vi "UHR-Fleezers Control (host) - 12.6.vi"() -> ()   [LabVIEW 2012] (continued)
                          n988 = call <vilib>:"Beep.vi"() -> ()  [unwired: 3 in, 9 out]
                          n989 = local write "Waiting"(FALSE ("Waiting")) -> ()
                          n990 = Increment(x=w1498) -> (x+1=w1497:u8)
                          n991 = case shown="\"Yank\"" w1500 {
                            tunnel: w1497 -> [_ _ w1507]
                            frame "Image" {
                              n992 = property on="Confocal Image" class="Bool (strict)"("Val(Sgnl)"=TRUE ("Value (Signaling)")) -> ()  [unwired: 2 in, 2 out]
                            }
                            frame "Alarm", Default {
                            }
                            frame "Yank" {
                              n993 = flat-sequence {
                                tunnel: w1507 -> [w1510]
                                tunnel: [w1509] -> w1506
                                tunnel: ["N Array El"] -> w1505
                                tunnel: w1506 -> [w1524]
                                tunnel: w1505 -> [w1520]
                                frame #0 {
                                n994 = Multiply(x="Yank Delay (s)", y=1000.0) -> (x*y=w1513:dbl)
                                n995 = Quotient & Remainder(x=w1510, y="N Array El") -> (x-y*floor(x/y)=w1509:u8)  [unwired: 1 out]
                                n996 = Wait (ms)(milliseconds to wait=w1513) -> ()  [unwired: 1 out]
                                }
                                frame #1 {
                                n997 = Random Number (0-1)() -> (number: 0 to 1=w1521:dbl)
                                n998 = Multiply(x=w1520, y=w1521) -> (x*y=w1519:dbl)
                                n999 = Round Toward -Infinity(1:w1519) -> (0:w1518:dbl)
                                n1000 = Select(t=w1518, s="Random Choice", f=w1524) -> (s? t:f=w1522:dbl)
                                n1001 = Select(t="Yank to Trap Delta (MHz)", s="Yank to which?", f="Yank to SP") -> (s? t:f=w1515:dbl[])
                                n1002 = Index Array(array=w1515, index=w1522) -> (element=w1525:dbl)
                                n1003 = case shown="False" "Yank to which?" {
                                tunnel: w1525 -> [w1526 w1552]
                                frame False {
                                n1004 = flat-sequence {
                                tunnel: w1526 -> [w1527]
                                frame #0 {
                                n1005 = property on="Trap Pos FB SP" class="DigNum (strict)"("Val(Sgnl)"=w1527) -> ()  [unwired: 2 in, 2 out]
                                }
                                frame #1 {
                                n1006 = Wait (ms)(milliseconds to wait=u32 700) -> ()  [unwired: 1 out]
                                }
                                frame #2 {
                                n1007 = local read "Action (%)"() -> (w1532:dbl)
                                n1008 = Absolute Value(x=w1532) -> (abs(x)=w1531:dbl)
                                n1009 = Greater?(x=w1531, y=70.0) -> (0:w1529:bool)
                                n1010 = property on="Remove Action Offset" class="Bool (strict)"("Val(Sgnl)"=w1529) -> ()  [unwired: 2 in, 2 out]
                                }
                                frame #3 {
                                n1011 = for {
                                N: 4 -> [_]
                                n1012 = flat-sequence {
                                frame #0 {
                                n1013 = Wait (ms)(milliseconds to wait=u32 500) -> ()  [unwired: 1 out]
                                }
                                frame #1 {
                                n1014 = local read "Action (%)"() -> (w1538:dbl)
                                n1015 = Absolute Value(x=w1538) -> (abs(x)=w1537:dbl)
                                n1016 = Greater?(x=w1537, y=70.0) -> (0:w1535:bool)
                                n1017 = property on="Remove Action Offset" class="Bool (strict)"("Val(Sgnl)"=w1535) -> ()  [unwired: 2 in, 2 out]
                                }
                                }
                                }
                                }
                                frame #4 {
                                n1018 = local read "Shift confocal"() -> (w1542:bool)
                                n1019 = local read "Mean"() -> (w1545:dbl)
                                n1020 = Greater?(x=w1545, y=11.0) -> (0:w1541:bool)
                                n1021 = Not(x=w1541) -> (.not. x?=w1540:bool)
                                n1022 = And(x=w1540, y=w1542) -> (x .and. y?=w1539:bool)
                                n1023 = And(x=w1541, y=w1542) -> (x .and. y?=w1543:bool)
                                n1024 = case shown="True" w1543 {
                                frame False {
                                }
                                frame True {
                                n1025 = local read "Confocal X 2 (V)"() -> (w1548:dbl)
                                n1026 = local read "Confocal Y 2 (V)"() -> (w1549:dbl)
                                n1027 = property on="AO2" class="Slide (strict)"("Val(Sgnl)"=w1548) -> ()  [unwired: 2 in, 2 out]
                                n1028 = property on="AO1" class="Slide (strict)"("Val(Sgnl)"=w1549) -> ()  [unwired: 2 in, 2 out]
                                }
                                }
                                n1029 = case shown="True" w1539 {
                                frame False {
                                }
                                frame True {
                                n1030 = local read "Confocal X 1 (V)"() -> (w1546:dbl)
                                n1031 = local read "Confocal Y 1 (V)"() -> (w1547:dbl)
                                n1032 = property on="AO1" class="Slide (strict)"("Val(Sgnl)"=w1547) -> ()  [unwired: 2 in, 2 out]
                                n1033 = property on="AO2" class="Slide (strict)"("Val(Sgnl)"=w1546) -> ()  [unwired: 2 in, 2 out]
                                }
                                }
                                }
                                frame #5 {
                                n1034 = Wait (ms)(milliseconds to wait=u32 1500) -> ()  [unwired: 1 out]
                                }
                                frame #6 {
                                n1035 = property on="Rem fb disp offset" class="Bool (strict)"("Val(Sgnl)"=TRUE ("Value (Signaling)")) -> ()  [unwired: 2 in, 2 out]
                                }
                                }
                                }
                                frame True {
                                n1036 = flat-sequence {
                                tunnel: w1552 -> [w1553]
                                frame #0 {
                                n1037 = property on="Trap Delta (MHz)" class="DigNum (strict)"("Val(Sgnl)"=w1553) -> ()  [unwired: 2 in, 2 out]
                                }
                                frame #1 {
                                n1038 = Wait (ms)(milliseconds to wait=u32 500) -> ()  [unwired: 1 out]
                                }
                                frame #2 {
                                n1039 = local read "Shift confocal"() -> (w1557:bool)
                                n1040 = local read "Mean"() -> (w1555:dbl)
                                n1041 = Greater?(x=w1555, y=11.0) -> (0:w1558:bool)
                                n1042 = Not(x=w1558) -> (.not. x?=w1559:bool)
                                n1043 = And(x=w1559, y=w1557) -> (x .and. y?=w1561:bool)
                                n1044 = And(x=w1558, y=w1557) -> (x .and. y?=w1560:bool)
                                n1045 = case shown="True" w1560 {
                                frame False {
                                }
                                frame True {
                                n1046 = local read "Confocal Y 2 (V)"() -> (w1565:dbl)
                                n1047 = local read "Confocal X 2 (V)"() -> (w1564:dbl)
                                n1048 = property on="AO1" class="Slide (strict)"("Val(Sgnl)"=w1565) -> ()  [unwired: 2 in, 2 out]
                                n1049 = property on="AO2" class="Slide (strict)"("Val(Sgnl)"=w1564) -> ()  [unwired: 2 in, 2 out]
                                }
                                }
                                n1050 = case shown="True" w1561 {
                                frame False {
                                }
                                frame True {
                                n1051 = local read "Confocal X 1 (V)"() -> (w1562:dbl)
                                n1052 = local read "Confocal Y 1 (V)"() -> (w1563:dbl)
                                n1053 = property on="AO2" class="Slide (strict)"("Val(Sgnl)"=w1562) -> ()  [unwired: 2 in, 2 out]
                                n1054 = property on="AO1" class="Slide (strict)"("Val(Sgnl)"=w1563) -> ()  [unwired: 2 in, 2 out]
                                }
                                }
                                }
                                }
                                }
                                }
                                }
                              }
                            }
                          }
                          n1055 = local read "Time (s)"() -> (w1499:dbl)
                          "Fl. High" <- TRUE ("Yanking")
                        }
                        frame #1 {
                          n1056 = local read "Auto F Reset"() -> (w1566:bool)
                          n1057 = case shown="True" w1566 {
                            tunnel: w1571 -> [_ w1575]
                            tunnel: w1570 -> [_ w1574]
                            tunnel: w1569 -> [_ w1573]
                            tunnel: w1567 -> [_ w1572]
                            frame False {
                            }
                            frame True {
                              n1058 = node-c288() -> (w1577:T23)  [unwired: 4 out]
                              n1059 = timed-loop {
                                timing: w1577 -> [_]
                                timing-out: [_] -> w1576
                                tunnel: w1575 -> [w1595]
                                tunnel: w1574 -> [w1594]
                                tunnel: w1573 -> [w1593]
                                tunnel: w1572 -> [w1592]
                                stop <- w1578 stop-if-true
                                n1060 = node-c288() -> ()  [unwired: 2 out]
                                n1061 = local read "Fl. Delta Thresh. (kHz)"() -> (w1586:dbl)
                                n1062 = local read "Fl. Triggered..."() -> (w1591:bool)
                                n1063 = local read "Delta Fl. 1"() -> (w1582:dbl)
                                n1064 = local read "Delta Fl. 2"() -> (w1580:dbl)
                                n1065 = local read "Stop All"() -> (w1589:bool)
                                n1066 = local read "APD to Watch"() -> (w1581:bool)
                                n1067 = Select(t=w1582, s=w1581, f=w1580) -> (s? t:f=w1579:dbl)
                                n1068 = Not(x=w1591) -> (.not. x?=w1590:bool)
                                n1069 = Multiply(x=w1586, y=1000.0) -> (x*y=w1585:dbl)
                                n1070 = Negate(x=w1585) -> (-x=w1584:dbl)
                                n1071 = Less?(x=w1579, y=w1584) -> (x < y?=w1588:bool)
                                n1072 = Compound Arithmetic op=OR(w1588, w1589, w1590, "Reset Force") -> (w1578:bool)
                                n1073 = case shown="True" w1578 {
                                tunnel: w1595 -> [_ w1610]
                                tunnel: w1594 -> [_ w1609]
                                tunnel: w1593 -> [_ w1599]
                                tunnel: w1592 -> [_ w1601]
                                frame False {
                                }
                                frame True {
                                n1074 = local read "Time (s)"() -> (w1600:dbl)
                                n1075 = case shown="\"Yank\"" w1609 {
                                tunnel: w1610 -> [_ w1613]
                                tunnel: w1601 -> [_ w1611]
                                frame "Image", Default {
                                }
                                frame "Yank" {
                                n1076 = flat-sequence {
                                tunnel: [w1619] -> w1614
                                tunnel: w1613 -> [w1619]
                                tunnel: [w1615] -> w1612
                                tunnel: w1611 -> [w1615]
                                tunnel: w1614 -> [w1622]
                                tunnel: w1612 -> [w1620]
                                frame #0 {
                                n1077 = local read "Yank Delay (s)"() -> (w1618:dbl)
                                n1078 = Multiply(x=w1618, y=1000.0) -> (x*y=w1616:dbl)
                                n1079 = Wait (ms)(milliseconds to wait=w1616) -> ()  [unwired: 1 out]
                                }
                                frame #1 {
                                n1080 = local read "Yank to which?"() -> (w1621:bool)
                                n1081 = case shown="False" w1621 {
                                tunnel: w1622 -> [_ w1649]
                                tunnel: w1620 -> [w1623 _]
                                frame False {
                                n1082 = flat-sequence {
                                tunnel: w1623 -> [w1624]
                                frame #0 {
                                n1083 = property on="Trap Pos FB SP" class="DigNum (strict)"("Val(Sgnl)"=w1624) -> ()  [unwired: 2 in, 2 out]
                                }
                                frame #1 {
                                n1084 = Wait (ms)(milliseconds to wait=u32 700) -> ()  [unwired: 1 out]
                                }
                                frame #2 {
                                n1085 = local read "Action (%)"() -> (w1629:dbl)
                                n1086 = Absolute Value(x=w1629) -> (abs(x)=w1628:dbl)
                                n1087 = Greater?(x=w1628, y=70.0) -> (0:w1626:bool)
                                n1088 = property on="Remove Action Offset" class="Bool (strict)"("Val(Sgnl)"=w1626) -> ()  [unwired: 2 in, 2 out]
                                }
                                frame #3 {
                                n1089 = for {
                                N: 4 -> [_]
                                n1090 = flat-sequence {
                                frame #0 {
                                n1091 = Wait (ms)(milliseconds to wait=u32 500) -> ()  [unwired: 1 out]
                                }
                                frame #1 {
                                n1092 = local read "Action (%)"() -> (w1635:dbl)
                                n1093 = Absolute Value(x=w1635) -> (abs(x)=w1634:dbl)
                                n1094 = Greater?(x=w1634, y=70.0) -> (0:w1632:bool)
                                n1095 = property on="Remove Action Offset" class="Bool (strict)"("Val(Sgnl)"=w1632) -> ()  [unwired: 2 in, 2 out]
                                }
                                }
                                }
                                }
                                frame #4 {
                                n1096 = local read "Shift confocal"() -> (w1640:bool)
                                n1097 = local read "Mean"() -> (w1642:dbl)
                                n1098 = Greater?(x=w1642, y=11.0) -> (0:w1639:bool)
                                n1099 = Not(x=w1639) -> (.not. x?=w1638:bool)
                                n1100 = And(x=w1639, y=w1640) -> (x .and. y?=w1637:bool)
                                n1101 = And(x=w1638, y=w1640) -> (x .and. y?=w1636:bool)
                                n1102 = case shown="True" w1637 {
                                frame False {
                                }
                                frame True {
                                n1103 = local read "Confocal Y 2 (V)"() -> (w1646:dbl)
                                n1104 = local read "Confocal X 2 (V)"() -> (w1645:dbl)
                                n1105 = property on="AO2" class="Slide (strict)"("Val(Sgnl)"=w1645) -> ()  [unwired: 2 in, 2 out]
                                n1106 = property on="AO1" class="Slide (strict)"("Val(Sgnl)"=w1646) -> ()  [unwired: 2 in, 2 out]
                                }
                                }
                                n1107 = case shown="True" w1636 {
                                frame False {
                                }
                                frame True {
                                n1108 = local read "Confocal X 1 (V)"() -> (w1643:dbl)
                                n1109 = local read "Confocal Y 1 (V)"() -> (w1644:dbl)
                                n1110 = property on="AO1" class="Slide (strict)"("Val(Sgnl)"=w1644) -> ()  [unwired: 2 in, 2 out]
                                n1111 = property on="AO2" class="Slide (strict)"("Val(Sgnl)"=w1643) -> ()  [unwired: 2 in, 2 out]
                                }
                                }
                                }
                                frame #5 {
                                n1112 = Wait (ms)(milliseconds to wait=u32 1500) -> ()  [unwired: 1 out]
                                }
                                frame #6 {
                                n1113 = property on="Rem fb disp offset" class="Bool (strict)"("Val(Sgnl)"=TRUE ("Value (Signaling)")) -> ()  [unwired: 2 in, 2 out]
                                }
                                }
                                }
                                frame True {
                                n1114 = flat-sequence {
                                tunnel: w1649 -> [w1650]
                                frame #0 {
                                n1115 = property on="Trap Delta (MHz)" class="DigNum (strict)"("Val(Sgnl)"=w1650) -> ()  [unwired: 2 in, 2 out]
                                }
                                frame #1 {
                                n1116 = Wait (ms)(milliseconds to wait=u32 500) -> ()  [unwired: 1 out]
                                }
                                frame #2 {
                                n1117 = local read "Shift confocal"() -> (w1656:bool)
                                n1118 = local read "Mean"() -> (w1658:dbl)
                                n1119 = Greater?(x=w1658, y=11.0) -> (0:w1655:bool)
                                n1120 = Not(x=w1655) -> (.not. x?=w1654:bool)
                                n1121 = And(x=w1655, y=w1656) -> (x .and. y?=w1653:bool)
                                n1122 = And(x=w1654, y=w1656) -> (x .and. y?=w1652:bool)
                                n1123 = case shown="True" w1653 {
                                frame False {
                                }
                                frame True {
                                n1124 = local read "Confocal Y 2 (V)"() -> (w1662:dbl)
                                n1125 = local read "Confocal X 2 (V)"() -> (w1661:dbl)
                                n1126 = property on="AO2" class="Slide (strict)"("Val(Sgnl)"=w1661) -> ()  [unwired: 2 in, 2 out]
                                n1127 = property on="AO1" class="Slide (strict)"("Val(Sgnl)"=w1662) -> ()  [unwired: 2 in, 2 out]
                                }
                                }
                                n1128 = case shown="True" w1652 {
                                frame False {
                                }
                                frame True {
                                n1129 = local read "Confocal Y 1 (V)"() -> (w1660:dbl)
                                n1130 = local read "Confocal X 1 (V)"() -> (w1659:dbl)
                                n1131 = property on="AO2" class="Slide (strict)"("Val(Sgnl)"=w1659) -> ()  [unwired: 2 in, 2 out]
                                n1132 = property on="AO1" class="Slide (strict)"("Val(Sgnl)"=w1660) -> ()  [unwired: 2 in, 2 out]
                                }
                                }
                                }
                                }
                                }
                                }
                                }
                                }
                                }
                                }
                                n1133 = local read "Messages"() -> (w1608:string)
                                n1134 = Subtract(x=w1600, y=w1599) -> (x-y=w1606:dbl)
                                "Duration (s)" <- w1606
                                n1135 = Number To Decimal String(number=w1606, width (-)=i16 0) -> (decimal integer string=w1604:string)
                                n1136 = Concatenate Strings(w1604, " s fluorescence event." ("string")) -> (w1602:string)
                                n1137 = call "Update messages.vi"("Message to add"=w1602, "Old message string"=w1608) -> ("New message string"=w1607:string)
                                n1138 = local write "Reset Force"(FALSE ("Reset Force")) -> ()
                                n1139 = local write "Waiting"(TRUE ("Waiting")) -> ()
                                n1140 = local write "Messages"(w1607) -> ()
                                n1141 = local write "Fl. High"(FALSE ("Fl. High")) -> ()
                                n1142 = call <vilib>:"Beep.vi"() -> ()  [unwired: 3 in, 9 out]
                                }
                                }
                                n1143 = node-c288() -> ()  [unwired: 2 out]
                              }
                              n1144 = node-c288(w1576) -> ()  [unwired: 1 out]
                            }
                          }
                        }
                      }
                      n1145 = local read "Trap Delta (MHz)"() -> (w1491:dbl)
                      n1146 = local read "Trap Pos FB SP"() -> (w1486:fxp<+/-,16,1>)
                    }
                  }
                }
                frame #1 {
                  n1147 = local read "Stop All"() -> (w1672:bool)
                  n1148 = local read "Fl. Triggered..."() -> (w1670:bool)
                  n1149 = Not(x=w1670) -> (.not. x?=w1671:bool)
                  n1150 = Or(x=w1671, y=w1672) -> (x .or. y?=w1669:bool)
                }
              }
              n1151 = case shown="True" w1263 {
                frame False {
                }
                frame True {
                  n1152 = local read "Confocal Y 1 (V)"() -> (w1273:dbl)
                  n1153 = local read "Confocal X 1 (V)"() -> (w1272:dbl)
                  n1154 = property on="AO2" class="Slide (strict)"("Val(Sgnl)"=w1272) -> ()  [unwired: 2 in, 2 out]
                  n1155 = property on="AO1" class="Slide (strict)"("Val(Sgnl)"=w1273) -> ()  [unwired: 2 in, 2 out]
                }
              }
              n1156 = case shown="True" w1263 {
                frame False {
                }
                frame True {
                  w1271 = FALSE ("Fl. High")
                  n1157 = local write "Waiting"(w1271) -> ()
                  n1158 = local write "Fl. High"(w1271) -> ()
                }
              }
              n1159 = node-c288() -> ()  [unwired: 2 out]
            }
            n1160 = node-c288(w1261) -> ()  [unwired: 1 out]
          }
        }
      }
      event "Stop All": Value Change {
        n1161 = event-data() -> ()  [unwired: 7 out]
        n1162 = local read "Stop All"() -> (w1677:bool)
      }
    }
    n1163 = node-c288() -> ()  [unwired: 2 out]
  }
  n1164 = timed-loop "Basic control parameters (all FPGA settings, other basic controls)" {
    tunnel: w16 -> [w1686]
    shift-right: [w1685] -> _
    shift-left: errorcluster {"status"=FALSE, "code"=0, "source"=""} ("error out") -> [w1684]
    tunnel: [w1683] -> _
    timing: w126 -> [_]
    timing-out: [_] -> w125
    tunnel: w99 -> [w1682]
    tunnel: w71 -> [w1681]
    tunnel: w70 -> [w1680]
    tunnel: w69 -> [w1679]
    tunnel: w68 -> [w1678]
    stop <- w1683 stop-if-true
    n1165 = node-c288() -> ()  [unwired: 2 out]
    n1166 = event shown="[4] \"Phase adj. (AI1)\", \"+ phase (AI1)\", \"- phase (AI1)\": Value Change" {
      selector: _ -> [_ _ _ _ _ _ _ _ _ _ _ _ _ _ _ _ _ _ _ _ _ _ _ _ _ _ _ _ _ _ _ _ _ _ _ _ _ _ _ _ _ _ _ _ _ _ _ _ _ _ _ _ _ _ _ _ _ _ _ _ _ _ _ _ _ _ _ _ _ _ _ _ _ _]
      dyn-events: _ -> [_ _ _ _ _ _ _ _ _ _ _ _ _ _ _ _ _ _ _ _ _ _ _ _ _ _ _ _ _ _ _ _ _ _ _ _ _ _ _ _ _ _ _ _ _ _ _ _ _ _ _ _ _ _ _ _ _ _ _ _ _ _ _ _ _ _ _ _ _ _ _ _ _ _]
      timeout: _ -> [_ _ _ _ _ _ _ _ _ _ _ _ _ _ _ _ _ _ _ _ _ _ _ _ _ _ _ _ _ _ _ _ _ _ _ _ _ _ _ _ _ _ _ _ _ _ _ _ _ _ _ _ _ _ _ _ _ _ _ _ _ _ _ _ _ _ _ _ _ _ _ _ _ _]
      tunnel: w1686 -> [w1727 _ _ _ w1765 _ w1787 _ _ _ _ w1853 _ _ w1896 w1902 w1909 w1914 w1987 _ w2003 w2028 w2049 w2070 w2090 w2119 w2145 w2148 w2152 w2247 w2252 w2290 _ w2325 w2329 w2340 w2344 w2348 _ w2356 _ _ _ _ _ _ _ _ _ _ _ _ _ _ _ _ _ w2734 _ w2751 _ w2758 w2776 _ w2783 w2791 w2806 w2822 w2828 _ w2837 _ w2856 _]
      tunnel: [w1726 _ _ _ w1755 _ w1786 _ _ w1818 _ w1832 _ _ w1895 w1898 w1908 w1911 w1981 _ w2002 w2027 w2047 w2068 w2088 w2113 w2143 _ w2150 w2245 w2250 w2288 _ w2323 w2327 w2331 w2342 w2346 _ w2354 _ _ _ _ _ _ _ _ _ _ _ _ _ _ _ _ _ w2732 _ _ _ _ w2773 _ _ _ _ _ _ _ _ _ _ _] -> w1685
      tunnel: w1684 -> [w1725 _ _ _ w1764 _ w1785 _ _ w1818 _ w1852 _ _ w1894 w1897 w1907 w1910 w1986 _ w2001 w2026 w2048 w2069 w2089 w2118 w2144 w2147 w2151 w2246 w2251 w2289 _ w2324 w2328 w2339 w2343 w2347 _ w2355 _ _ _ _ _ _ _ _ _ _ _ _ _ _ _ _ _ w2733 _ w2750 _ w2757 w2775 _ w2782 w2790 w2805 w2821 w2827 _ w2836 _ w2855 _]
      tunnel: [_ _ _ _ _ _ _ _ _ w1817 _ _ _ _ _ _ _ _ _ _ _ _ _ _ _ _ _ _ _ _ _ _ _ _ _ _ _ _ _ _ _ _ _ _ _ _ _ _ _ _ _ _ _ _ _ _ _ _ _ _ _ _ _ _ _ _ _ _ _ _ _ _ _ _] -> w1683
      tunnel: [_ _ _ _ _ _ _ "Round T1 X" _ _ _ _ _ _ _ _ _ _ _ _ _ _ _ _ _ _ _ _ _ _ _ _ _ _ _ _ _ _ _ _ _ _ _ _ _ _ _ _ _ _ _ _ _ _ _ _ _ _ _ _ _ _ _ _ _ _ _ _ _ _ _ _ _ _] -> _
      tunnel: [_ _ _ "Adjust Scale\nto Mean" _ _ _ _ _ _ _ _ _ _ _ _ _ _ _ _ _ _ _ _ _ _ _ _ "Test ttrig" _ _ _ _ _ _ _ _ _ _ _ _ _ _ _ _ _ _ "Flush Sample" "Flush Pump 3" "Flush Pump 1" "Clear Volume" _ _ _ _ _ _ _ _ _ _ _ _ _ _ _ _ _ _ _ _ _ _ _] -> _
      tunnel: [_ _ _ _ _ _ _ _ "Round T2 X" _ "Delayed Interlace Start" _ _ _ _ _ _ _ _ _ _ _ _ _ _ _ _ _ _ _ _ _ _ _ _ _ _ _ _ _ _ _ _ _ _ _ _ _ _ _ _ _ _ _ _ _ _ _ _ _ _ _ _ _ _ _ _ _ _ _ _ _ _ _] -> _
      tunnel: w1682 -> [_ _ _ _ _ _ _ _ _ _ _ _ _ _ _ _ _ _ _ _ _ _ _ _ _ _ _ _ _ _ _ _ _ _ _ _ _ _ _ _ _ _ _ w2513 w2520 w2527 w2532 w2541 _ _ w2647 _ _ _ _ _ _ _ _ _ _ _ _ _ _ _ _ _ _ _ _ _ _ _]
      tunnel: w1681 -> [_ _ _ _ _ _ _ _ _ _ _ _ _ _ _ _ _ _ _ _ _ _ _ _ _ _ _ _ _ _ _ _ _ _ _ _ _ _ _ _ _ w2430 _ _ _ _ _ _ w2585 _ _ w2653 _ w2662 _ w2676 _ _ _ _ _ _ _ _ _ _ _ _ _ _ _ _ _ _]
      tunnel: w1680 -> [_ _ _ _ _ _ _ _ _ _ _ _ _ _ _ _ _ _ _ _ _ _ _ _ _ _ _ _ _ _ _ _ _ _ _ _ _ _ _ _ _ _ _ _ _ _ _ _ _ _ _ _ _ _ _ _ _ _ _ _ _ _ _ _ _ _ _ _ _ _ _ _ _ _]
      tunnel: w1679 -> [_ _ _ _ _ _ _ _ _ _ _ _ _ _ _ _ _ _ _ _ _ _ _ _ _ _ _ _ _ _ _ _ _ _ _ _ _ _ _ _ w2367 _ _ _ _ _ _ _ _ w2615 _ _ w2658 _ w2669 _ w2701 _ _ _ _ _ _ _ _ _ _ _ _ _ _ _ _ _]
      tunnel: w1678 -> [_ _ _ _ _ _ _ _ _ _ _ _ _ _ _ _ _ _ _ _ _ _ _ _ _ _ _ _ _ _ _ _ _ _ _ _ _ _ _ _ _ _ _ _ _ _ _ _ _ _ _ _ _ _ _ _ _ _ _ _ _ _ _ _ _ _ _ _ _ _ _ _ _ _]
      event "AI Count (ticks)", "Sets to FIFO (Traps)", "Save ave N", "FPGA Ave.", "# Samples/channel", "N sets to save": Value Change {
        # "So that if 'Save ave N' is updated, the AOD scanning code updates too."
        n1167 = event-data() -> ()  [unwired: 6 out]
        n1168 = local read "AI Count (ticks)"() -> (w1709:u16)
        n1169 = Unbundle By Name("Sets to FIFO (Traps)") -> ("Set 1"=w1692:bool, "Set 2"=w1691:bool, "Set 3"=w1690:bool)
        n1170 = Boolean To (0,1)(Boolean="Sets to FIFO (Traps)") -> (0, 1=w1717:cluster{"Set 1":i16, "Set 2":i16, "Set 3":i16})
        n1171 = xnode "Read/Write Control"("FPGA VI Reference In"=w1727, "error in"=w1725, "ai count"=w1709, "Set 1"=w1692, "Set 2"=w1691, "Set 3"=w1690, "N of AI1 Int Acq Sets"="N Acq Sets (Traps + Fl.)") -> ("error out"=w1726:errorcluster)  [unwired: 1 out]
        n1172 = Cluster To Array(cluster=w1717) -> (array=w1716:i16[])
        n1173 = To Unsigned Long Integer(number=w1716) -> (unsigned 32bit integer=w1698:u32[])
        n1174 = local read "Scan steps (AOD)"() -> (w1718:u64)
        n1175 = Multiply(x=w1709, y="N Acq Sets (Traps + Fl.)") -> (x*y=w1707:u16)
        n1176 = Divide(x=40000000.0, y=w1709) -> (x/y=w1701:dbl)
        "AI rate (Hz)" <- w1701
        "Ave. Rate (Hz)" <- w1701
        n1177 = Add Array Elements(numeric array=w1698) -> (sum=w1710:u32)
        "Trap Sets" <- w1710
        n1178 = Reciprocal(x=w1701) -> (1/x=→"Ave. Period (s)":dbl)
        n1179 = property on="Scan steps (AOD)" class="DigNum (strict)"("Val(Sgnl)"=w1718) -> ()  [unwired: 2 in, 2 out]
        n1180 = Divide(x=w1701, y="N Acq Sets (Traps + Fl.)") -> (x/y=w1722:dbl)
        "Data Rate (Hz)" <- w1722
        n1181 = Reciprocal(x=w1722) -> (1/x=→"Data Period (s)":dbl)
        n1182 = local read "Save ave N"() -> (w1721:dbl)
        n1183 = Divide(x=w1722, y=w1721) -> (x/y=w1720:dbl)
        "Save Data Rate (Hz)" <- w1720
        n1184 = Reciprocal(x=w1720) -> (1/x=→"Save Data Period (s)":dbl)
        n1185 = Multiply(x=w1707, y="# Samples/trap") -> (x*y=w1705:u32)
        "Counts/DMA" <- w1705
        n1186 = property on="Trap Disp. Downsample" class="DigNum (strict)"("Maximum"="# Samples/trap") -> ()  [unwired: 2 in, 2 out]
        n1187 = Multiply(x=w1710, y="# Samples/trap") -> (x*y=w1699:u32)
        "# Samples/channel" <- w1699
        n1188 = Multiply(x=w1699, y=u32 8) -> (x*y=→"Trap AI Elements/DMA read":u32)
        n1189 = local read "APD Int. Count"() -> (w1706:u32)
        n1190 = Multiply(x=w1699, y=u32 3) -> (x*y=→"Trap Pos Elements/DMA read":u32)
        n1191 = Divide(x=w1705, y=w1706) -> (x/y=w1696:dbl)
        "APD Samples/FIFO Acq." <- w1696
        n1192 = Divide(x=w1705, y=40000000.0) -> (x/y=w1703:dbl)
        "DMA Update Period (s)" <- w1703
        n1193 = local read "Number of APDs"() -> (w1689:u8)
        n1194 = Multiply(x=w1689, y=w1696) -> (x*y=→"APD Elements/DMA read":dbl)
        n1195 = property on="APD Disp. Downsample" class="DigNum (strict)"("Maximum"=w1696) -> ()  [unwired: 2 in, 2 out]
        n1196 = local read "N sets to save"() -> (w1715:u32)
        n1197 = Multiply(x=w1703, y=w1715) -> (x*y=→"Total Time (s)":dbl)
        "FPGA Averaging" <- FALSE ("FPGA Averaging")
      }
      event "Remove Offset": Value Change {
        n1198 = event-data() -> ()  [unwired: 7 out]
        n1199 = local write "Remove Offset"(FALSE ("Remove Offset")) -> ()
        n1200 = local read "Bead Mean (nm)"() -> (w1729:dbl)
        n1201 = local read "Offset (nm)"() -> (w1730:dbl)
        n1202 = Add(x=w1729, y=w1730) -> (x+y=w1728:dbl)
        n1203 = local write "Offset (nm)"(w1728) -> ()
        n1204 = disable-structure shown="Disabled" {
          frame Disabled {
            n1205 = local read "Bead Mean (nm)"() -> (w1735:dbl)
            n1206 = Add(y=w1735) -> (x=w1734:dbl, x+y=w1733:dbl)
            n1207 = Subtract(x=w1735, y=w1734) -> (x-y=w1732:dbl)
            n1208 = property on="Bead Separation" class="WFChart (strict)"("YScale.Minimum"=w1732) -> ()  [unwired: 2 in, 2 out]
            n1209 = property on="Bead Separation" class="WFChart (strict)"("YScale.Maximum"=w1733) -> ()  [unwired: 2 in, 2 out]
          }
          frame Enabled {
          }
        }
      }
      event "Detector Type": Value Change {
        n1210 = event-data() -> ()  [unwired: 7 out]
        n1211 = local read "AI labels"() -> (w1736:string[])
        n1212 = property on="High Res. Display" class="Ring (strict)"("Strings []"=w1736) -> ()  [unwired: 2 in, 2 out]
        n1213 = Build Array (concatenate)(w1736, "none") -> (w1737:string[])
        n1214 = property on="FFT 1 Choice 1" class="Ring (strict)"("Strings []"=w1737) -> ()  [unwired: 2 in, 2 out]
        n1215 = property on="FFT 1 Choice 2" class="Ring (strict)"("Strings []"=w1737) -> ()  [unwired: 2 in, 2 out]
        n1216 = property on="FFT 2 Choice 1" class="Ring (strict)"("Strings []"=w1737) -> ()  [unwired: 2 in, 2 out]
        n1217 = property on="FFT 2 Choice 2" class="Ring (strict)"("Strings []"=w1737) -> ()  [unwired: 2 in, 2 out]
        n1218 = Bundle("APD 1", "APD 2") -> (w1740:cluster{string, string})  [unwired: 1 out]
        n1219 = Cluster To Array(cluster=w1740) -> (array=w1738:string[])
        n1220 = Build Array (concatenate)(w1738, w1737) -> (w1742:string[])
        n1221 = Array Size(array=w1742) -> (size(s)=w1743:i32)
        n1222 = property on="Signals to Plot" class="LstBox (strict)"("Item Names"=w1742) -> ()  [unwired: 2 in, 2 out]
        n1223 = property on="Signals to Plot" class="LstBox (strict)"("Number of Rows"=w1743) -> ()  [unwired: 2 in, 2 out]
        n1224 = property on="All Signals" class="WFChart (strict)"("LegNumRows"=w1743) -> ()  [unwired: 2 in, 2 out]
      }
      event "Adjust Scale\nto Mean": Value Change {
        n1225 = event-data() -> ()  [unwired: 7 out]
        n1226 = local read "APD 1 Rate (Hz)"() -> (w1752:dbl)
        n1227 = Multiply(x=1000.0, y="Above (kHz)") -> (x*y=w1750:dbl)
        n1228 = Multiply(x=1000.0, y="Below (kHz)") -> (x*y=w1748:dbl)
        n1229 = Add(x=w1750, y=w1752) -> (x+y=w1745:dbl)
        n1230 = Subtract(x=w1752, y=w1748) -> (x-y=w1746:dbl)
        n1231 = property on="APD Chart" class="WFChart (strict)"("YScale.Minimum"=w1746) -> ()  [unwired: 2 in, 2 out]
        n1232 = property on="APD Chart" class="WFChart (strict)"("YScale.Maximum"=w1745) -> ()  [unwired: 2 in, 2 out]
      }
      event "Phase adj. (AI1)", "+ phase (AI1)", "- phase (AI1)": Value Change {
        n1233 = event-data() -> ()  [unwired: 7 out]
        n1234 = Negate(x="Phase adj. (AI1)") -> (-x=w1762:i16)
        n1235 = Select(t=w1762, s="- phase (AI1)", f="Phase adj. (AI1)") -> (s? t:f=w1761:i16)
        n1236 = xnode "Read/Write Control"("FPGA VI Reference In"=w1765, "error in"=w1764, "Phase count adjustment"=w1761) -> ("FPGA VI Reference Out"=w1760:T20, "error out"=w1759:errorcluster)  [unwired: 1 in]
        n1237 = Or(x="- phase (AI1)", y="+ phase (AI1)") -> (x .or. y?=w1756:bool)
        n1238 = xnode "Read/Write Control"("FPGA VI Reference In"=w1760, "error in"=w1759, "+ phase"=w1756) -> ("error out"=w1755:errorcluster)  [unwired: 1 in, 1 out]
      }
      event "Signals to Plot": Double Click {
        w1768 = u32 9868950 ("Color Box")
        n1239 = event-data() -> ("Row"=w1770:i32)  [unwired: 9 out]
        n1240 = property on="All Signals" class="WFChart (strict)"("Active Plot"=w1770) -> (error out=w1781:errorcluster)  [unwired: 2 in, 1 out]
        n1241 = property on="All Signals" class="WFChart (strict)" props=["Plot", "Visible?", "Plot", "Plot Color"](error in=w1781) -> (error out=w1780:errorcluster, "Plot.Visible?"=w1779:bool)  [unwired: 1 in, 2 out]
        n1242 = Select(t=FALSE ("Plot.Visible"), s=w1779, f=TRUE ("Plot.Visible")) -> (s? t:f=w1774:bool)
        n1243 = property on="All Signals" class="WFChart (strict)"(error in=w1780, "Plot.Visible?"=w1774) -> (error out=w1776:errorcluster)  [unwired: 1 in, 1 out]
        n1244 = property on="All Signals" class="WFChart (strict)"(error in=w1776) -> (error out=w1771:errorcluster, "Plot.Plot Color"=w1775:u32)  [unwired: 1 in, 1 out]
        n1245 = property on="Signals to Plot" class="LstBox (strict)"(error in=w1771, "Active Row"=w1770) -> (error out=w1769:errorcluster)  [unwired: 1 in, 1 out]
        n1246 = Select(t=w1775, s=w1774, f=u32 0) -> (s? t:f=w1772:u32)
        n1247 = property on="Signals to Plot" class="LstBox (strict)"(error in=w1769, "CellFontColor"=w1772, "SelColor"=w1768, "CellBG"=w1768, "CellFontSize"=u32 20 ("Active Row:Cell Font:Size"), "CellFontBold"=TRUE ("Active Row:Cell Font:Bold")) -> ()  [unwired: 1 in, 2 out]
      }
      event "BD 1 Frequency 1 (MHz)", "BD 1 Frequency 2 (MHz)", "BD 1 Frequency 3 (MHz)", "BD 2 Frequency 1 (MHz)", "BD 2 Frequency 2 (MHz)", "BD 2 Frequency 3 (MHz)", "Trap Delta (MHz)": Value Change {
        n1248 = event-data() -> ("CtlRef"=w1784:refnum<vi>)  [unwired: 6 out]
        n1249 = control-ref of="Trap Delta (MHz)"() -> (w1783:refnum<vi>)
        n1250 = Equal?(x=w1783, y=w1784) -> (x = y?=w1782:bool)
        n1251 = case shown="False" "Oscillate Set 1" {
          tunnel: w1787 -> [w1807 _]
          tunnel: [w1806 w1810] -> w1786
          tunnel: w1785 -> [w1805 w1810]
          tunnel: w1782 -> [w1790 _]
          frame False {
            n1252 = local read "BD 1 Frequency 2 (MHz)"() -> (w1794:dbl)
            n1253 = local read "BD 1 Frequency 1 (MHz)"() -> (w1792:dbl)
            n1254 = Subtract(x=w1794, y="Trap Delta (MHz)") -> (x-y=w1791:dbl)
            n1255 = Select(t=w1791, s=w1790, f=w1792) -> (s? t:f=w1789:dbl)
            n1256 = local read "Y RF Frequency Limits (MHz)"() -> (w1795:T16)
            n1257 = local read "X RF Frequency Limits (MHz)"() -> (w1796:T16)
            n1258 = local read "BD 1 Frequency 3 (MHz)"() -> (w1808:dbl)
            n1259 = local write "BD 1 Frequency 1 (MHz)"(w1789) -> ()
            n1260 = local read "BD 2 Frequency 1 (MHz)"() -> (w1799:dbl)
            n1261 = local read "BD 2 Frequency 2 (MHz)"() -> (w1798:dbl)
            n1262 = local read "BD 2 Frequency 3 (MHz)"() -> (w1809:dbl)
            n1263 = call "set RF board frequency - interlace.vi"("Board 2 Frequency Limits"=w1795, "Board 1 Frequency Limits"=w1796, "error in"=w1805, "FPGA VI Reference In"=w1807, "Board 2 Frequency 3 (MHz)"=w1809, "Board 1 Frequency 3 (MHz)"=w1808, "Board 2 Frequency 2 (MHz)"=w1798, "Board 2 Frequency 1 (MHz)"=w1799, "Board 1 Frequency 2 (MHz)"=w1794, "Board 1 Frequency 1  (MHz)"=w1789) -> ("error out"=w1806:errorcluster)  [unwired: 1 out]
            n1264 = Subtract(x=w1799, y=w1798) -> (x-y=w1803:dbl)
            n1265 = Subtract(x=w1789, y=w1794) -> (x-y=w1804:dbl)
            n1266 = Square(x=w1803) -> (x^2=w1801:dbl)
            n1267 = Square(x=w1804) -> (x^2=w1802:dbl)
            n1268 = Add(x=w1802, y=w1801) -> (x+y=w1800:dbl)
            n1269 = Square Root(x=w1800) -> (sqrt(x)=w1797:dbl)
            n1270 = local write "Trap Delta (MHz)"(w1797) -> ()
            n1271 = property on="Initial delta (MHz)" class="DigNum (strict)"("Val(Sgnl)"=w1797) -> ()  [unwired: 2 in, 2 out]
          }
          frame True {
          }
        }
      }
      event "Round T1 X": Value Change {
        n1272 = event-data() -> ()  [unwired: 7 out]
        n1273 = local read "BD 1 Frequency 1 (MHz)"() -> (w1813:dbl)
        n1274 = Round To Nearest(number=w1813) -> (nearest integer value=w1812:dbl)
        n1275 = property on="BD 1 Frequency 1 (MHz)" class="DigNum (strict)"("Val(Sgnl)"=w1812) -> ()  [unwired: 2 in, 2 out]
      }
      event "Round T2 X": Value Change {
        n1276 = event-data() -> ()  [unwired: 7 out]
        n1277 = local read "BD 1 Frequency 2 (MHz)"() -> (w1815:dbl)
        n1278 = Round To Nearest(number=w1815) -> (nearest integer value=w1814:dbl)
        n1279 = property on="BD 1 Frequency 2 (MHz)" class="DigNum (strict)"("Val(Sgnl)"=w1814) -> ()  [unwired: 2 in, 2 out]
      }
      event "Stop All": Value Change {
        n1280 = event-data() -> ()  [unwired: 7 out]
        n1281 = local read "Stop All"() -> (w1817:bool)
      }
      event "Delayed Interlace Start": Value Change {
        n1282 = event-data() -> ()  [unwired: 7 out]
        n1283 = flat-sequence {
          frame #0 {
            n1284 = Multiply(x="Delay to Interlace (s)", y=1000.0) -> (x*y=w1820:dbl)
            n1285 = Wait (ms)(milliseconds to wait=w1820) -> ()  [unwired: 1 out]
          }
          frame #1 {
            n1286 = property on="Laser interlacing mode" class="RadioBtnsControl (strict)"("Val(Sgnl)"=enum32{"Laser ON", "Laser OFF", "Interlace"}."Interlace" ("Value (Signaling)")) -> ()  [unwired: 2 in, 2 out]
          }
        }
      }
      event "BD 1 Amplitude 1 (%)", "BD 1 Amplitude 2 (%)", "BD 1 Amplitude 3 (%)", "BD 2 Amplitude 1 (%)", "BD 2 Amplitude 2 (%)", "BD 2 Amplitude 3 (%)", "Trap 1 ON", "Trap 2 ON", "Trap 3 ON", "Feedback On/Off", "All FB On/Off": Value Change {
        w1844 = i16 1 ("f")
        n1287 = event-data() -> ()  [unwired: 7 out]
        n1288 = local write "Trap 1 (ON/OFF)"("Trap 1 ON") -> ()
        n1289 = local write "Trap 2 (ON/OFF)"("Trap 2 ON") -> ()
        n1290 = Boolean To (0,1)(Boolean="Trap 3 ON") -> (0, 1=w1845:i16)
        n1291 = Boolean To (0,1)(Boolean="Trap 1 ON") -> (0, 1=w1846:i16)
        n1292 = Boolean To (0,1)(Boolean="Trap 2 ON") -> (0, 1=w1847:i16)
        n1293 = Select(t=w1847, s="Trap ON/OFF X or Y Amp?", f=w1844) -> (s? t:f=w1842:i16)
        n1294 = Select(t=w1846, s="Trap ON/OFF X or Y Amp?", f=w1844) -> (s? t:f=w1843:i16)
        n1295 = Select(t=w1845, s="Trap ON/OFF X or Y Amp?", f=w1844) -> (s? t:f=w1841:i16)
        n1296 = Select(t=w1844, s="Trap ON/OFF X or Y Amp?", f=w1847) -> (s? t:f=w1839:i16)
        n1297 = Select(t=w1844, s="Trap ON/OFF X or Y Amp?", f=w1846) -> (s? t:f=w1840:i16)
        n1298 = Select(t=w1844, s="Trap ON/OFF X or Y Amp?", f=w1845) -> (s? t:f=w1838:i16)
        n1299 = And(x="All FB On/Off", y="Feedback On/Off") -> (x .and. y?=w1836:cluster{"Set 1":bool, "Set 2":bool})
        n1300 = local read "BD 1 Amplitude 1 (%)"() -> (w1856:dbl)
        n1301 = local read "BD 1 Amplitude 2 (%)"() -> (w1855:dbl)
        n1302 = local read "BD 1 Amplitude 3 (%)"() -> (w1854:dbl)
        n1303 = Unbundle By Name(w1836) -> ("Set 1"=w1831:bool, "Set 2"=w1828:bool)
        n1304 = local read "Y RF Amplitude Limits (%)"() -> (w1824:T16)
        n1305 = local read "X RF Amplitude Limits (%)"() -> (w1825:T16)
        n1306 = local read "BD 2 Amplitude 1 (%)"() -> (w1857:dbl)
        n1307 = local read "BD 2 Amplitude 2 (%)"() -> (w1858:dbl)
        n1308 = local read "BD 2 Amplitude 3 (%)"() -> (w1859:dbl)
        n1309 = And(x="Trap 2 ON", y=w1828) -> (x .and. y?=w1826:bool)
        n1310 = And(x="Trap 1 ON", y=w1831) -> (x .and. y?=w1829:bool)
        n1311 = Multiply(x=w1843, y=w1856) -> (x*y=w1851:dbl)
        n1312 = Multiply(x=w1855, y=w1842) -> (x*y=w1849:dbl)
        n1313 = Multiply(x=w1854, y=w1841) -> (x*y=w1850:dbl)
        n1314 = Multiply(x=w1857, y=w1840) -> (x*y=w1860:dbl)
        n1315 = Multiply(x=w1858, y=w1839) -> (x*y=w1861:dbl)
        n1316 = Multiply(x=w1859, y=w1838) -> (x*y=w1862:dbl)
        n1317 = call "set RF board amplitude - interlace.vi"("Board 2 Amplitude Limits"=w1824, "Board 1 Amplitude Limits"=w1825, "error in"=w1852, "FPGA VI Reference In"=w1853, "Board 2 Amplitude 3 (%)"=w1862, "Board 1 Amplitude 3 (%)"=w1850, "Board 2 Amplitude 2 (%)"=w1861, "Board 2 Amplitude 1 (%)"=w1860, "Board 1 Amplitude 2 (%)"=w1849, "Board 1 Amplitude 1 (%)"=w1851) -> ("error out"=w1833:errorcluster, "FPGA VI Reference Out"=w1834:T20)
        n1318 = xnode "Read/Write Control"("FPGA VI Reference In"=w1834, "error in"=w1833, "FB On/Off Set 1"=w1829, "FB On/Off Set 2"=w1826) -> ("error out"=w1832:errorcluster)  [unwired: 1 out]
      }
      event "Load parameters": Value Change {
        n1319 = event-data() -> ()  [unwired: 7 out]
        n1320 = property on="Saved AOD Raster Scan Parameter Sets" class="Arr (strict)"() -> ("Index Values"=w1873:u32[])  [unwired: 2 in, 2 out]
        n1321 = Index Array(array=w1873, index=0) -> (element=w1870:u32)
        n1322 = local write "Load parameters"(FALSE ("Load parameters")) -> ()
        n1323 = Index Array(array="Saved AOD Raster Scan Parameter Sets", index=w1870) -> (element=w1869:T30)
        n1324 = Unbundle By Name(w1869) -> ("Scan Range AOD (nm) 2"=w1868:dbl, "Step Size AOD (nm) 2"=w1867:dbl, "Scan Speed AOD (nm/s) 2"=w1866:dbl, "Number of scans (AOD) 2"=w1865:u16)
        n1325 = flat-sequence {
          tunnel: w1868 -> [w1876]
          tunnel: w1867 -> [w1875]
          tunnel: w1866 -> [w1874]
          tunnel: w1865 -> [w1877]
          frame #0 {
            n1326 = local write "Scan Speed (nm/s)"(w1874) -> ()
            n1327 = local write "Scan Range (nm)"(w1876) -> ()
            n1328 = local write "Step Size (nm)"(w1875) -> ()
          }
          frame #1 {
            n1329 = property on="Number of F/B Scans (AOD)" class="DigNum (strict)"("Val(Sgnl)"=w1877) -> ()  [unwired: 2 in, 2 out]
          }
        }
      }
      event "Trap 1 (ON/OFF)", "Trap 2 (ON/OFF)": Value Change {
        n1330 = event-data() -> ()  [unwired: 7 out]
        n1331 = property on="Trap 2 ON" class="Bool (strict)"("Val(Sgnl)"="Trap 2 (ON/OFF)") -> ()  [unwired: 2 in, 2 out]
        n1332 = property on="Trap 1 ON" class="Bool (strict)"("Val(Sgnl)"="Trap 1 (ON/OFF)") -> ()  [unwired: 2 in, 2 out]
      }
      event "DIO count 1 (ticks)", "DIO count 2 (ticks)", "DIO count 3 (ticks)", "Interlace", "Number Interlace Sets", "Not-Interlacing Set": Value Change {
        n1333 = event-data() -> ()  [unwired: 7 out]
        n1334 = local read "DIO count 3 (ticks)"() -> (w1890:u16)
        n1335 = local read "DIO count 1 (ticks)"() -> (w1892:u16)
        n1336 = local read "DIO count 2 (ticks)"() -> (w1891:u16)
        n1337 = To Unsigned Byte Integer(number="Not-Interlacing Set") -> (unsigned 8bit integer=w1881:u8)
        n1338 = Add(x=w1881, y=u8 1) -> (x+y=w1885:u8)
        n1339 = xnode "Read/Write Control"("FPGA VI Reference In"=w1896, "error in"=w1894, "DIO count 1 (ticks)"=w1892, "DIO count 2 (ticks)"=w1891, "DIO count 3 (ticks)"=w1890, "Interlace ON/OFF"="Interlace", "Number Interlace Cycles"="Number Interlace Sets", "Interlace Off Parameters"=w1885) -> ("error out"=w1895:errorcluster)  [unwired: 1 out]
        n1340 = Build Array(w1892, w1891, w1890) -> (w1883:u16[])
        n1341 = Split 1D Array(array=w1883, index="Number Interlace Sets") -> (first subarray=w1893:u16[])  [unwired: 1 out]
        n1342 = Index Array(array=w1883, index=w1881) -> (element=w1882:u16)
        n1343 = Add Array Elements(numeric array=w1893) -> (sum=w1887:u16)
        n1344 = Select(t=w1887, s="Interlace", f=w1882) -> (s? t:f=→"Total Counts (ticks)":u16)
      }
      event "Reset Feedback": Value Change {
        n1345 = event-data() -> ()  [unwired: 7 out]
        n1346 = Unbundle By Name("Reset Feedback") -> ("Set 1"=w1900:bool, "Set 2"=w1899:bool)
        n1347 = xnode "Read/Write Control"("FPGA VI Reference In"=w1902, "error in"=w1897, "FB Reset Set 1"=w1900, "FB Reset Set 2"=w1899) -> ("error out"=w1898:errorcluster)  [unwired: 1 out]
      }
      event "Trap Intensity PID Gains": Value Change {
        n1348 = event-data() -> ()  [unwired: 7 out]
        n1349 = Unbundle By Name("Trap Intensity PID Gains") -> ("proportional gain (Kc)"=w1905:i16, "integral gain (Kc*Ts/Ti)"=w1904:i16, "derivative gain (Kc*Td/Ts)"=w1903:i16)
        n1350 = xnode "Read/Write Control"("FPGA VI Reference In"=w1909, "error in"=w1907, "P1"=w1905, "I1"=w1904, "D1"=w1903) -> ("error out"=w1908:errorcluster)  [unwired: 1 out]
      }
      event "AI2 to Setpoint", "Setpoints (V)": Value Change {
        n1351 = event-data() -> ()  [unwired: 7 out]
        n1352 = xnode "Read/Write Control"("FPGA VI Reference In"=w1914, "error in"=w1910) -> ("FPGA VI Reference Out"=w1913:T20, "error out"=w1912:errorcluster, "AI2 Y Sum Set 1"=w1921:i16, "AI2 Y Sum Set 2"=w1920:i16)
        n1353 = Cluster To Array(cluster="AI2 to Setpoint") -> (array=w1924:bool[])
        n1354 = local read "AI2 (V)"() -> (w1922:cluster{"Set 1":dbl, "Set 2":dbl})
        n1355 = Or Array Elements(Boolean array=w1924) -> (logical OR=w1925:bool)
        n1356 = Bundle By Name(cluster=w1922, "Set 1"=w1921, "Set 2"=w1920) -> (w1919:cluster{"Set 1":dbl, "Set 2":dbl})
        n1357 = Divide(x=w1919, y=3276.7) -> (x/y=w1918:cluster{"Set 1":dbl, "Set 2":dbl})
        "AI2 (V)" <- w1918
        n1358 = case shown="True" w1925 {
          tunnel: [w1928 w1945] -> w1917
          tunnel: "AI2 to Setpoint" -> [_ w1941]
          tunnel: "Setpoints (V)" -> [w1929 w1944]
          tunnel: w1918 -> [_ w1938]
          frame False {
            n1359 = Multiply(x=3276.7, y=w1929) -> (x*y=w1930:cluster{"Set 1":dbl, "Set 2":dbl})
            n1360 = To Word Integer(number=w1930) -> (16bit integer=w1928:cluster{"Set 1":i16, "Set 2":i16})
          }
          frame True {
            n1361 = Unbundle By Name(w1938) -> ("Set 1"=w1937:dbl, "Set 2"=w1936:dbl)
            n1362 = Unbundle By Name(w1944) -> ("Set 1"=w1943:dbl, "Set 2"=w1942:dbl)
            n1363 = Unbundle By Name(w1941) -> ("Set 1"=w1940:bool, "Set 2"=w1939:bool)
            n1364 = Select(t=w1937, s=w1940, f=w1943) -> (s? t:f=w1935:dbl)
            n1365 = Select(t=w1936, s=w1939, f=w1942) -> (s? t:f=w1934:dbl)
            n1366 = Bundle By Name(cluster=w1944, "Set 1"=w1935, "Set 2"=w1934) -> (w1932:cluster{"Set 1":dbl, "Set 2":dbl})
            n1367 = local write "Setpoints (V)"(w1932) -> ()
            n1368 = Multiply(x=3276.7, y=w1932) -> (x*y=w1933:cluster{"Set 1":dbl, "Set 2":dbl})
            n1369 = To Word Integer(number=w1933) -> (16bit integer=w1945:cluster{"Set 1":i16, "Set 2":i16})
          }
        }
        n1370 = Unbundle By Name(w1917) -> ("Set 1"=w1916:i16, "Set 2"=w1915:i16)
        n1371 = xnode "Read/Write Control"("FPGA VI Reference In"=w1913, "error in"=w1912, "FB Setpoint Set 1"=w1916, "FB Setpoint Set 2"=w1915) -> ("error out"=w1911:errorcluster)  [unwired: 1 out]
      }
      event "+ phase (GI)", "- phase (GI)", "+ phase (GI) 2", "- phase (GI) 2", "+ phase (RI)", "- phase (RI)", "+ phase (Green FB)", "- phase (Green FB)": Value Change {
        n1372 = event-data() -> ()  [unwired: 7 out]
        n1373 = Or(x="+ phase (GI)", y="- phase (GI)") -> (x .or. y?=w1980:bool)
        n1374 = Negate(x="Phase adj. (GI)") -> (-x=w1985:i16)
        n1375 = Select(t=w1985, s="+ phase (GI)", f="Phase adj. (GI)") -> (s? t:f=w1984:i16)
        n1376 = Or(x="+ phase (GI) 2", y="- phase (GI) 2") -> (x .or. y?=w1971:bool)
        n1377 = Negate(x="Phase adj. (GI) 2") -> (-x=w1976:i16)
        n1378 = Select(t=w1976, s="+ phase (GI) 2", f="Phase adj. (GI) 2") -> (s? t:f=w1972:i16)
        n1379 = Negate(x="Phase adj. (RI)") -> (-x=w1970:i16)
        n1380 = Or(x="+ phase (RI)", y="- phase (RI)") -> (x .or. y?=w1966:bool)
        n1381 = Select(t=w1970, s="+ phase (RI)", f="Phase adj. (RI)") -> (s? t:f=w1965:i16)
        n1382 = Or(x="+ phase (Green FB)", y="- phase (Green FB)") -> (x .or. y?=w1959:bool)
        n1383 = Negate(x="Phase adj. (Green FB)") -> (-x=w1964:i16)
        n1384 = Select(t=w1964, s="+ phase (Green FB)", f="Phase adj. (Green FB)") -> (s? t:f=w1960:i16)
        n1385 = Negate(x="Phase adj. (BI AO)") -> (-x=w1958:i16)
        n1386 = Or(x="+ phase (BI AO)", y="- phase (BI AO)") -> (x .or. y?=w1948:bool)
        n1387 = Select(t=w1958, s="+ phase (BI AO)", f="Phase adj. (BI AO)") -> (s? t:f=w1950:i16)
        n1388 = Negate(x="Phase adj. (BI DO)") -> (-x=w1954:i16)
        n1389 = Or(x="+ phase (BI DO)", y="- phase (BI DO)") -> (x .or. y?=w1947:bool)
        n1390 = Select(t=w1954, s="+ phase (BI DO)", f="Phase adj. (BI DO)") -> (s? t:f=w1949:i16)
        n1391 = xnode "Read/Write Control"("FPGA VI Reference In"=w1987, "error in"=w1986, "Phase count adjustment (GI)"=w1984, "Phase count adjustment (GI) 2"=w1972, "Phase count adjustment (RI)"=w1965, "Phase count adjustment (Green FB)"=w1960, "Phase count adjustment (BI AO)"=w1950, "Phase count adjustment (BI D)"=w1949) -> ("FPGA VI Reference Out"=w1982:T20, "error out"=w1983:errorcluster)
        n1392 = xnode "Read/Write Control"("FPGA VI Reference In"=w1982, "error in"=w1983, "+ phase (GI)"=w1980, "+ phase (GI) 2"=w1971, "+ phase (RI)"=w1966, "+ phase (Green FB)"=w1959, "+ phase (BI AO)"=w1948, "+ phase (BI D)"=w1947) -> ("error out"=w1981:errorcluster)  [unwired: 1 out]
      }
      event "Green Laser ON/OFF", "Red Laser ON/OFF", "Blue Laser ON/OFF": Value Change {
        # "This loop shouldn't be initialized.  The main 'laser ON' settings should dominate and set the others."
        n1393 = event-data() -> ()  [unwired: 7 out]
        n1394 = property on="Red Laser ON" class="Bool (strict)"("Val(Sgnl)"="Red Laser ON/OFF") -> ()  [unwired: 2 in, 2 out]
        n1395 = property on="Blue Laser ON" class="Bool (strict)"("Val(Sgnl)"="Blue Laser ON/OFF") -> ()  [unwired: 2 in, 2 out]
